vi "edit io channel.vi"(6 "user event":T2, 7 "instance identifier":string, 8 "error in":errorcluster, 9 "line":T1, 10 "engine configuration in":refnum<class "engine configuration.lvclass">, 11 "Profibus Module configuration in":refnum<class "Profibus Module configuration.lvclass">) -> (0 "error out":errorcluster, 2 "engine configuration out":refnum<class "engine configuration.lvclass">, 3 "Profibus Module configuration out":refnum<class "Profibus Module configuration.lvclass">)   [LabVIEW 2013, in "Profibus Module editor node.lvclass"]
uses:
  Profibus Module editor node.lvclass
  <vilib>/CEF_TreeControl/Node/UserEventRef.ctl
  <vilib>/CEF_TreeControl/Controls/EventCluster.ctl
  <vilib>/NI/Module Execution Interface/Engine Configuration/engine configuration.lvclass
  <vilib>/NI/TBM Modules/Profibus/configuration/Profibus Module configuration.lvclass
  table line.ctl
  <vilib>/NI/TBM Modules/Profibus/channel/Profibus channel.lvclass
  <vilib>/NI/Tag Bus/tag/tag descriptor.lvclass/tag descriptor.ctl
  <vilib>/CEF_TreeControl/NISE_CEF_TreeControl.lvlib
  <vilib>/NI/Tag Bus/tag/tag descriptor.lvclass
  <vilib>/CEF_TreeControl/Node/NISE_CEF_Node.lvclass
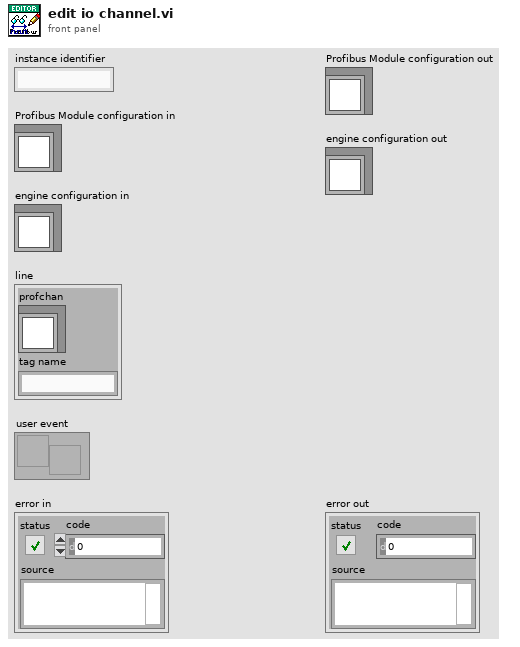
[diagram p1: front panel]
types:
  T1 = typedef "Profibus Module editor node.lvclass/table line.ctl" = cluster{"profchan":refnum<class "Profibus channel.lvclass">, "tag name":string}
  T2 = typedef "NISE_CEF_Node.lvclass/UserEventRef.ctl" = refnum<user-event>
  T3 = typedef "NISE_CEF_TreeControl.lvlib/EventCluster.ctl" = cluster{"command":string, "data":string}
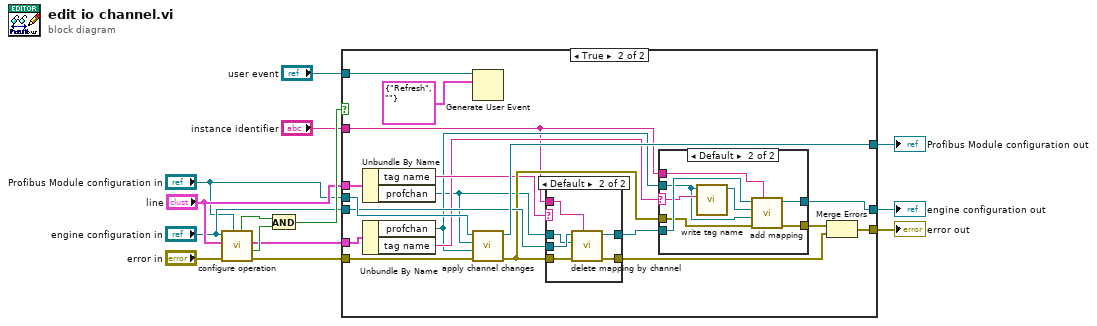
[diagram p0: block diagram]
diagram:
  n1 = call "configure operation.vi"("owner ID"="Profibus Module configuration in", "error in"="error in", "line item in"="line", "engine configuration in"="engine configuration in") -> ("error out"=w6:errorcluster, "success"=w10:bool, "line item out"=w7:T1, "changed"=w9:bool)  [unwired: 4 in]
  n2 = And(x=w9, y=w10) -> (x .and. y?=w11:bool)
  n3 = case shown="True" w11 {
    tunnel: [w16 w26] -> w4
    tunnel: [w17 w24] -> w13
    tunnel: "engine configuration in" -> [w17 w25]
    tunnel: w6 -> [w16 w34]
    tunnel: w7 -> [_ w31]
    tunnel: "line" -> [_ w35]
    tunnel: "Profibus Module configuration in" -> [w15 w36]
    tunnel: [w15 w30] -> w12
    tunnel: "instance identifier" -> [_ w18]
    tunnel: "user event" -> [_ w32]
    frame False {
    }
    frame True {
      n4 = Unbundle By Name(w35) -> ("tag name"=w22:string, "profchan"=w19:refnum<class "Profibus channel.lvclass">)
      n5 = Unbundle By Name(w31) -> ("profchan"=w20:refnum<class "Profibus channel.lvclass">, "tag name"=w21:string)
      n6 = Generate User Event(user event=w32, event data cluster=T3 {"command"="Refresh", "data"=""} ("event data")) -> ()  [unwired: 2 in, 2 out]
      n7 = call <vilib>:"apply channel changes.vi"("error in"=w34, "new"=w20, "old"=w19, "Profibus Module configuration in"=w36) -> ("error out"=w23:errorcluster, "Profibus Module configuration out"=w30:refnum<class "Profibus Module configuration.lvclass">)  [unwired: 6 in]
      n8 = case shown="Default" w22 {
        tunnel: w18 -> [_ w54]
        tunnel: w25 -> [w48 w53]
        tunnel: [w48 w52] -> w27
        tunnel: [w47 w51] -> w28
        tunnel: w23 -> [w47 w50]
        tunnel: w19 -> [_ w49]
        frame "" {
        }
        frame Default {
          n9 = call <vilib>:"delete mapping by channel.vi"("owner ID"=w54, "error in"=w50, "channel"=w49, "engine configuration in"=w53) -> ("error out"=w51:errorcluster, "engine configuration out"=w52:refnum<class "engine configuration.lvclass">)  [unwired: 6 in]
        }
      }
      n10 = case shown="Default" w21 {
        selector: w21 -> [_ w40]
        tunnel: w27 -> [w38 w46]
        tunnel: [w38 w45] -> w24
        tunnel: [w37 w44] -> w29
        tunnel: w23 -> [w37 w43]
        tunnel: w18 -> [_ w42]
        tunnel: w20 -> [_ w39]
        frame "" {
        }
        frame Default {
          n11 = call <vilib>:"write tag name.vi"("name"=w40, "system tag in"=w39) -> ("system tag out"=w41:refnum<class "Profibus channel.lvclass">)  [unwired: 8 in, 1 out]
          n12 = call <vilib>:"add mapping.vi"("owner ID"=w42, "error in"=w43, "channel"=w39, "tag descriptor"=w41, "engine configuration"=w46) -> ("error out"=w44:errorcluster, "engine configuration out"=w45:refnum<class "engine configuration.lvclass">)  [unwired: 5 in]
        }
      }
      n13 = Merge Errors(w29, w28) -> (w26:errorcluster)
    }
  }
  "engine configuration out" <- w13
  "Profibus Module configuration out" <- w12
  "error out" <- w4
